vi "Recuperation de donnees.vi"(9 "Est-ce un string?":bool, 10 "Array in":string[][](array[string]), 11 "Refnum in":T1) -> (1 "Array":dbl[](array[numeric]), 3 "String out":string[](array[string]))   [LabVIEW 2017]
uses:
  <vilib>/Utility/config.llb/Config Data RefNum.ctl
  <vilib>/Utility/config.llb/Read Key (Double).vi
  <vilib>/Utility/config.llb/Read Key (String).vi
  <vilib>/Utility/config.llb/NI_LVConfig.lvlib
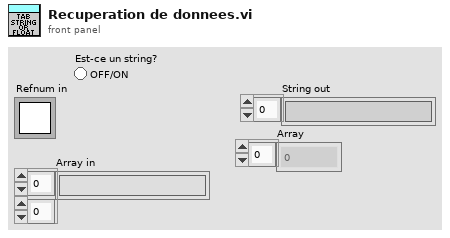
[diagram p1: front panel]
types:
  T1 = typedef "NI_LVConfig.lvlib/Config Data RefNum.ctl" = refnum<k1>
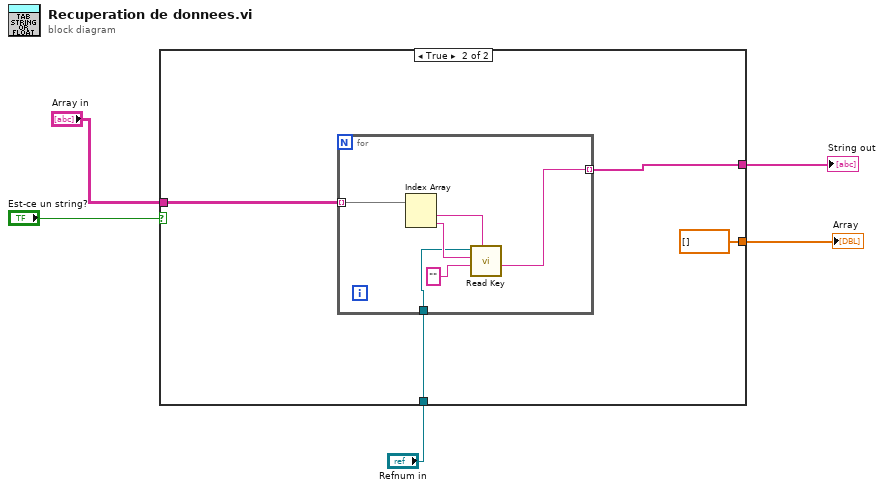
[diagram p0: block diagram]
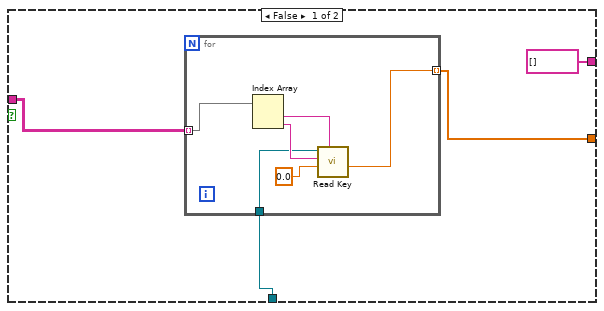
[diagram p2: hidden frame]
diagram:
  n1 = case shown="True" "Est-ce un string?" {
    tunnel: "Array in" -> [w8 w19]
    tunnel: [string[] [] w18] -> w3
    tunnel: "Refnum in" -> [w7 w17]
    tunnel: [w6 dbl[] []] -> w1
    frame False {
      n2 = for {
        tunnel: w8 -> [w13] mode=indexing
        tunnel: w7 -> [w12]
        tunnel: [w11] -> w6 mode=indexing
        n3 = Index Array(array=w13) -> (element #1=w15:string, element #2=w14:string)  [unwired: 2 in]
        n4 = call-poly <vilib>:"Read Key.vi"("section"=w15, "default value"=0.0, "key"=w14, "refnum"=w12) -> ("value"=w11:dbl)  [unwired: 4 in, 3 out]
      }
    }
    frame True {
      n5 = for {
        tunnel: [w23] -> w18 mode=indexing
        tunnel: w19 -> [w21] mode=indexing
        tunnel: w17 -> [w20]
        n6 = Index Array(array=w21) -> (element #1=w25:string, element #2=w24:string)  [unwired: 2 in]
        n7 = call-poly <vilib>:"Read Key.vi"("section"=w25, "default value"="", "key"=w24, "refnum"=w20) -> ("value"=w23:string)  [unwired: 4 in, 3 out]
      }
    }
  }
  "String out" <- w3
  "Array" <- w1
